vi "MotionMagicDrive.vi"(1 "Enable Vision Y":bool, 4 "X offset":dbl format="%#_13g", 5 "High gear?":bool, 6 "Y offset":dbl format="%#_13g", 7 "Enable Vision X":bool, 8 "error in (no error)":errorcluster, 9 "Y Axis":dbl, 10 "X Axis":dbl, 11 "Pod Drive in":refnum<class "Pod Drive.lvclass">) -> (0 "error out":errorcluster, 3 "Pod Drive out":refnum<class "Pod Drive.lvclass">)   [LabVIEW 2018, in "Drive.lvlib" / "Pod Drive.lvclass"]
doc: "This VI alows you to swich between motion magic GoTo and Closed Loop"
uses:
  Pod Drive.lvclass
  Controls/Mode.ctl
  Drive.lvclass
panel:
  in  "Xmultiplyer":dbl=70.0 format="%#_13g"
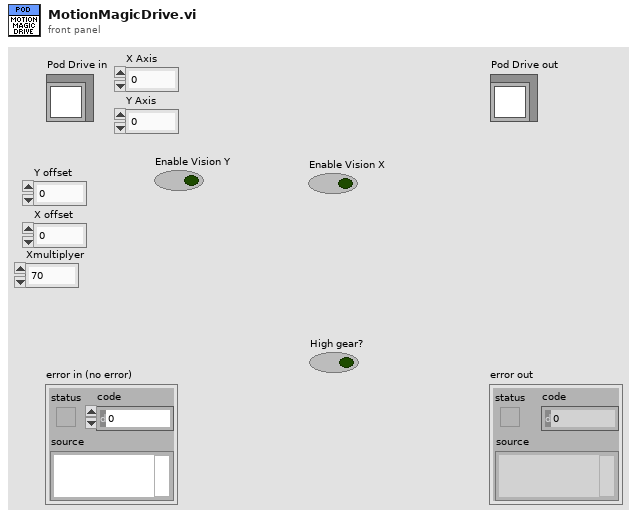
[diagram p1: front panel]
types:
  T1 = typedef "Drive.lvlib/Pod Drive.lvclass/Mode.ctl" = enum16{"ClosedLoop", "MotionMagic"}
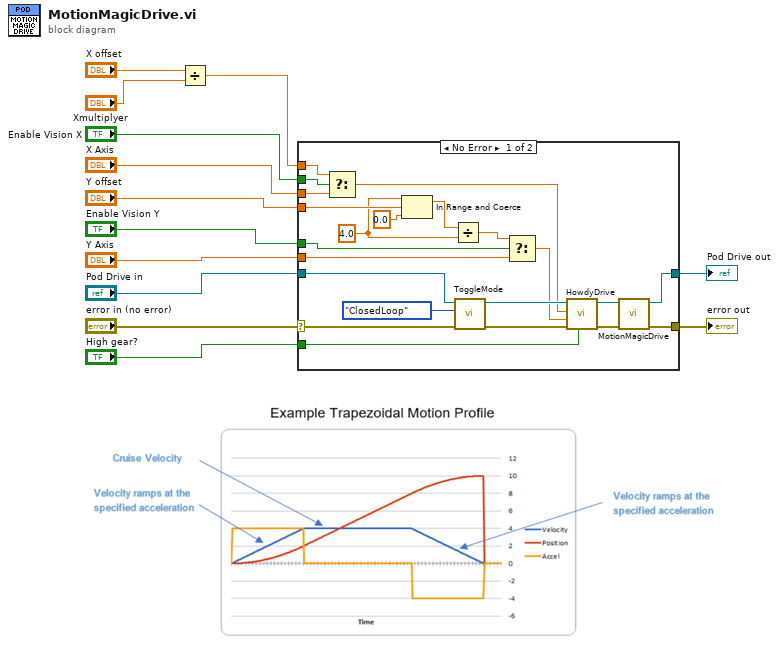
[diagram p0: block diagram]
diagram:
  n1 = Divide(x="X offset", y="Xmultiplyer") -> (x/y=w4:dbl)
  n2 = case shown="No Error" "error in (no error)" {
    selector: "error in (no error)" -> [w31 w36]
    tunnel: [w35 w36] -> w13
    tunnel: [w34 w37] -> w12
    tunnel: "Pod Drive in" -> [w30 w37]
    tunnel: "Enable Vision X" -> [w24 _]
    tunnel: "X Axis" -> [w28 _]
    tunnel: w4 -> [w23 _]
    tunnel: "Y Axis" -> [w20 _]
    tunnel: "High gear?" -> [w27 _]
    tunnel: "Enable Vision Y" -> [w19 _]
    tunnel: "Y offset" -> [w17 _]
    frame No Error {
      w15 = 4.0 ("upper limit")
      n3 = Select(t=w23, s=w24, f=w28) -> (s? t:f=w22:dbl)
      n4 = In Range and Coerce(upper limit=w15, x=w17, lower limit=0.0) -> (coerced(x)=w16:dbl)  [unwired: 1 out]
      n5 = Divide(x=w16, y=w15) -> (x/y=w14:dbl)
      n6 = call-dynamic "ToggleMode.vi"("error in (no error)"=w31, "Mode"=Mode."ClosedLoop" ("ClosedLoopOrMotionMagic"), "Pod Drive in"=w30) -> ("error out"=w26:errorcluster, "Pod Drive out"=w29:refnum<class "Pod Drive.lvclass">)  [unwired: 7 in]
      n7 = Select(t=w14, s=w19, f=w20) -> (s? t:f=w21:dbl)
      n8 = call-dynamic "HowdyDrive.vi"("HighGear?"=w27, "error in (no error)"=w26, "Y"=w21, "X"=w22, "Pod Drive in"=w29) -> ("error out"=w32:errorcluster, "Pod Drive out"=w33:refnum<class "Pod Drive.lvclass">)  [unwired: 5 in]
      n9 = call-parent "MotionMagicDrive.vi"("error in (no error)"=w32, "Drive in"=w33) -> ("error out"=w35:errorcluster, "Drive out"=w34:refnum<class "Pod Drive.lvclass">)  [unwired: 8 in]
    }
    frame Error {
    }
  }
  "error out" <- w13
  "Pod Drive out" <- w12
